vi "Cleanup.vi"(8 "error in (no error)":errorcluster, 11 "SOL-Server in":refnum<class "SOL-Server.lvclass">) -> (0 "error out":errorcluster)   [LabVIEW 2020, in "Summer of LabVIEW.lvlib" / "SOL-Server.lvclass"]
uses:
  SOL-Server.lvclass
  SOL-Server.lvclass/SOL-Server.ctl
  <vilib>/IlluminatedG/IG HTTP Server/HTTP Server/Server/Server.lvclass
  SQLite/SQLite.lvclass
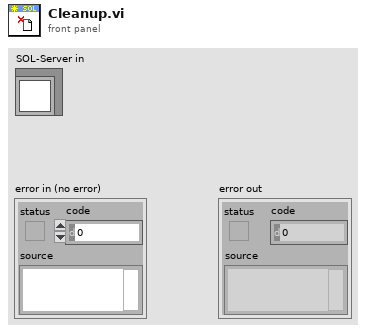
[diagram p1: front panel]
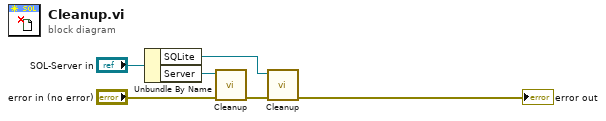
[diagram p0: block diagram]
diagram:
  n1 = Unbundle By Name("SOL-Server in") -> ("SQLite"=w2:refnum<class "SQLite.lvclass">, "Server"=w5:refnum<class "Server.lvclass">)
  n2 = call <vilib>:"Cleanup.vi"("error in (no error)"="error in (no error)", "Server in"=w5) -> ("error out"=w3:errorcluster)  [unwired: 9 in]
  n3 = call <vilib>:"Cleanup.vi"("error in (no error)"=w3, "SQLite in"=w2) -> ("error out"=→"error out":errorcluster)  [unwired: 9 in]
